vi "CAN_OBD仿真器.vi"() -> ()   [LabVIEW 2018]
doc: "This example demonstrates frame streaming input using an NI-XNET Frame Input session. \n\nThis example can run against any output example, assuming you have a properly terminated CAN cable connected to two CAN ports.\n\nIf you have no database aliases on your system, the example automatically loads the nixnet_example database."
uses:
  <vilib>/xnet/xnet.llb/XNET Frame CAN.ctl
  <vilib>/xnet/xnet.llb/XNET Frame Type CAN.ctl
  <vilib>/xnet/xnet.llb/XNET Create Session (Frame Input Stream).vi
  <vilib>/xnet/xnet.llb/XNET Create Session (Frame Output Stream).vi
  <vilib>/xnet/xnet.llb/XNET Read (Frame CAN).vi
  <vilib>/xnet/xnet.llb/XNET Write (Frame CAN).vi
  <resource>/objmgr/xnet.rc
panel:
  in  "车速":u8(slide) scale=0.0..255.0
  in  "引擎转速":u16(slide) scale=0.0..20000.0
  out "data":T1[](array[typedef]) {"payload" format="%x"; "timestamp" format="%<%.7X\n%x>T"; "type" items=["CAN Data"=0, "CAN Remote"=1, "CAN Bus Error"=2, "CAN 2.0 Data"=8, "CAN FD Data"=16, "CAN FD+BRS Data"=24, "J1939 Data"=192, "Delay"=224, "Log Trigger"=225, "Start Trigger"=226]; "identifier" format="%x"}
  in  "Number of Frames to Display":i32=15
  in  "Hex Display":bool=TRUE
  in  "BaudRate":u32=500000
  out "Frames":string[][](table)
  in  "Select Interface":refnum<k21>="CAN2"
  in  "stop":bool
  # "Overview: Demonstrates the use of the CAN streaming frame input session.\nRequirements: LabVIEW, NI-XNET\nInstructions:\n1. Ensure that you are have connected the selected CAN port to another CAN interface outputting data. This example can be used with any CAN output example.\n2. Run the VI"
  # "If a cluster is selected, the cluster's baudrate will be used.  If the :memory: cluster is selected, a baudrate must be provided."
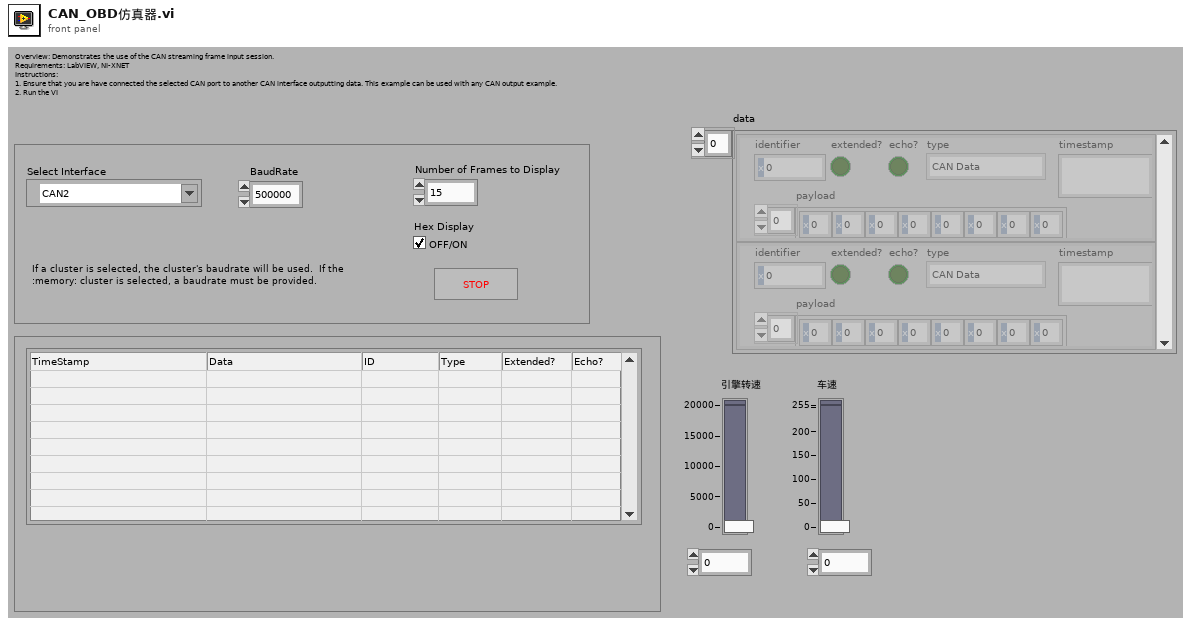
[diagram p1: front panel]
types:
  T1 = typedef "XNET Frame CAN.ctl" = cluster{"timestamp":timestamp, "payload":u8[], "identifier":u32, "type":T2, "extended?":bool, "echo?":bool}
  T2 = typedef "XNET Frame Type CAN.ctl" = u8
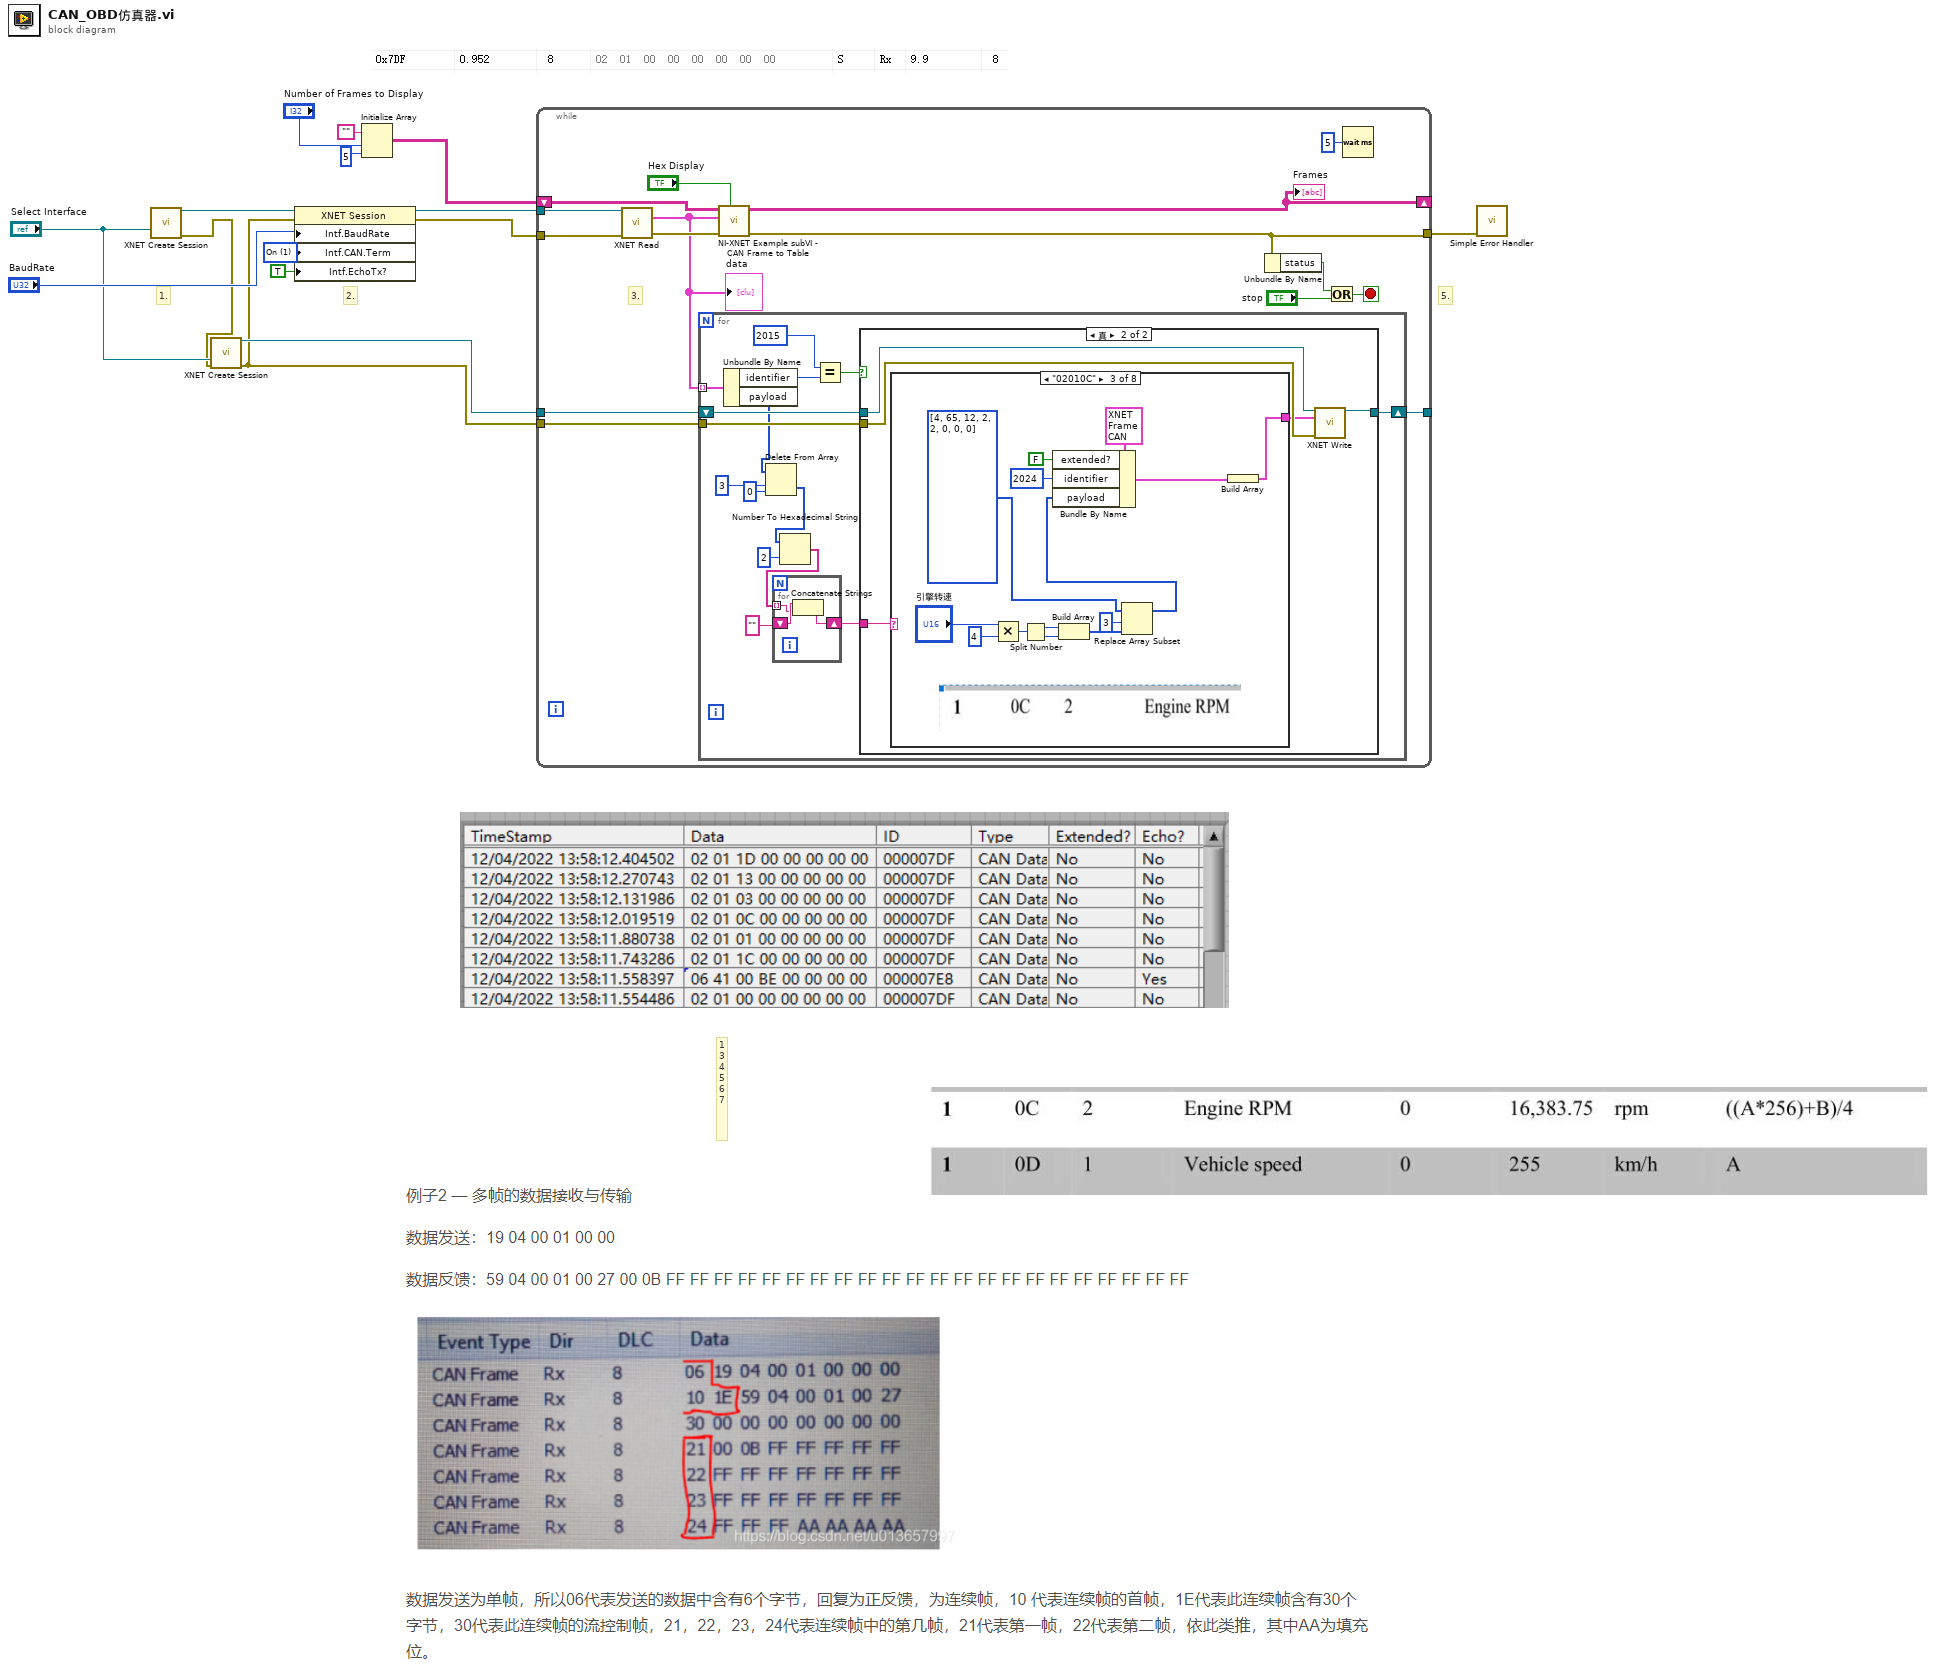
[diagram p0: block diagram]
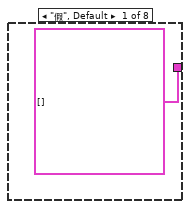
[diagram p3: hidden frame]
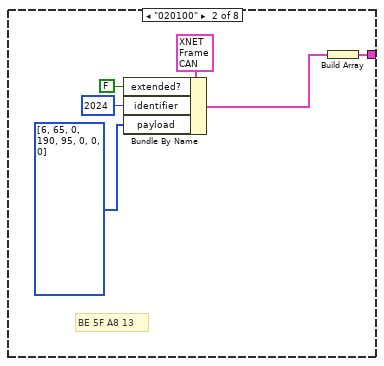
[diagram p4: hidden frame]
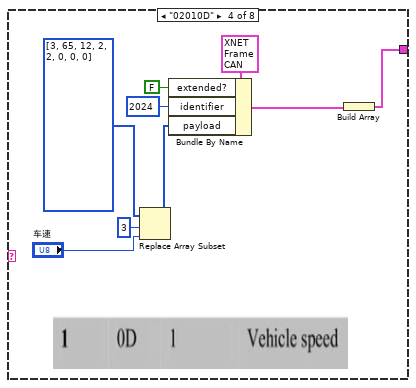
[diagram p5: hidden frame]
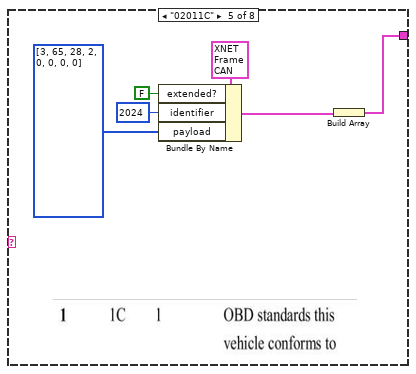
[diagram p6: hidden frame]
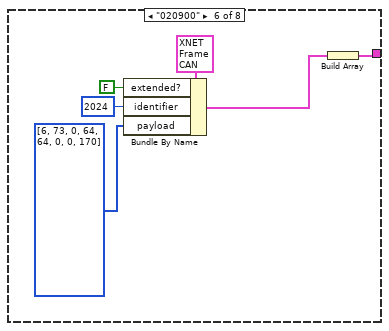
[diagram p7: hidden frame]
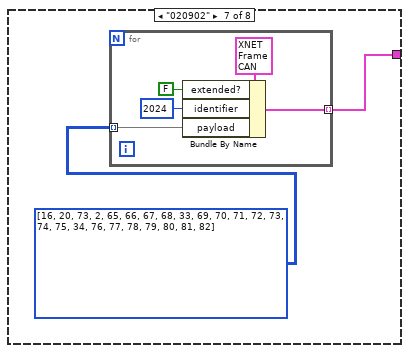
[diagram p8: hidden frame]
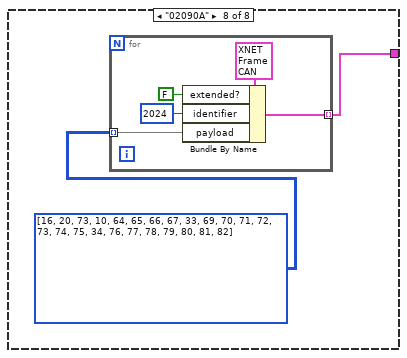
[diagram p9: hidden frame]
diagram:
  w6 = u32 1 items=["Off", "On"] ("Interface:CAN:Termination")
  # "1\n3\n4\n5\n6\n7"
  # "2."
  # "5."
  # "1."
  n1 = call-poly <vilib>:"XNET Create Session.vi"("interface"="Select Interface") -> ("session out"=w14:refnum<k21>, "error out"=w4:errorcluster)  [unwired: 2 in, 11 out]
  n2 = call-poly <vilib>:"XNET Create Session.vi"("interface"="Select Interface", "error in (no error)"=w4) -> ("session out"=w3:refnum<k21>, "error out"=w2:errorcluster)  [unwired: 1 in, 11 out]
  n3 = property class="XNET Session"(reference=w14, error in=w2, "Intf.BaudRate"="BaudRate", "Intf.CAN.Term"=w6, "Intf.EchoTx?"=TRUE ("Interface:Echo Transmit?")) -> (reference out=w13:refnum<k21>, error out=w11:errorcluster)
  n4 = Initialize Array("", "Number of Frames to Display", 5 ("Dimension Size")) -> (w7:string[][])
  n5 = while {
    tunnel: w13 -> [w30]
    tunnel: w11 -> [w29]
    tunnel: [w22] -> w15
    shift-right: [w24] -> _
    shift-left: w7 -> [w25]
    tunnel: w3 -> [w18]
    tunnel: w2 -> [w17]
    tunnel: [w16] -> _
    stop <- w26 stop-if-true
    # "3."
    n6 = call-poly <vilib>:"XNET Read.vi"("session in"=w30, "error in (no error)"=w29) -> ("data"=w19:T1[], "error out"=w23:errorcluster)  [unwired: 12 out]
    "data" <- w19
    n7 = for {
      tunnel: w19 -> [w45] mode=indexing
      tunnel: w17 -> [w43]
      shift-right: [w42] -> w16
      shift-left: w18 -> [w44]
      n8 = Unbundle By Name(w45) -> ("identifier"=w40:u32, "payload"=w34:u8[])
      n9 = Delete From Array(array=w34, length=3 ("长度"), index=0 ("索引")) -> (deleted portion=w33:u8[])  [unwired: 1 out]
      n10 = Number To Hexadecimal String(1:i16 2 ("宽度(-)"), 2:w33) -> (0:w38:string[])
      n11 = for {
        shift-right: [w48] -> w35
        shift-left: "" -> [w47]
        tunnel: w38 -> [w46] mode=indexing
        n12 = Concatenate Strings(w47, w46) -> (w48:string)
      }
      n13 = Equal?(x=u32 2015 ("y"), y=w40) -> (x = y?=w41:bool)
      n14 = case shown="真" w41 {
        tunnel: w44 -> [w49 w50]
        tunnel: w43 -> [_ w54]
        tunnel: [w49 w51] -> w42
        tunnel: w35 -> [_ w53]
        frame False {
        }
        frame True {
          n15 = case shown="\"02010C\"" w53 {
            tunnel: [T1[] [] w56 w71 w80 w86 w91 w98 w104] -> w52
            frame "假", Default {
            }
            frame "020100" {
              # "BE 5F A8 13"
              n16 = Bundle By Name(cluster=T1 {"timestamp"=timestamp(0 s since 1904-01-01), "payload"=[], "identifier"=0, "type"=0, "extended?"=FALSE, "echo?"=FALSE} ("CAN frame"), "extended?"=FALSE, "identifier"=u32 2024, "payload"=u8[] [6, 65, 0, 190, 95, 0, 0, 0]) -> (w60:T1)
              n17 = Build Array(w60) -> (w56:T1[])
            }
            frame "02010C" {
              n18 = Multiply(x="引擎转速", y=u16 4) -> (x*y=w69:u16)
              n19 = Split Number(x=w69) -> (hi(x)=w68:u8, lo(x)=w67:u8)
              n20 = Build Array(w68, w67) -> (w66:u8[])
              n21 = Replace Array Subset(array=u8[] [4, 65, 12, 2, 2, 0, 0, 0] ("payload"), new element=w66, index=3 ("索引")) -> (w62:u8[])
              n22 = Bundle By Name(cluster=T1 {"timestamp"=timestamp(0 s since 1904-01-01), "payload"=[], "identifier"=0, "type"=0, "extended?"=FALSE, "echo?"=FALSE} ("CAN frame"), "extended?"=FALSE, "identifier"=u32 2024, "payload"=w62) -> (w72:T1)
              n23 = Build Array(w72) -> (w71:T1[])
            }
            frame "02010D" {
              n24 = Replace Array Subset(array=u8[] [3, 65, 12, 2, 2, 0, 0, 0] ("payload"), new element="车速", index=3 ("索引")) -> (w76:u8[])
              n25 = Bundle By Name(cluster=T1 {"timestamp"=timestamp(0 s since 1904-01-01), "payload"=[], "identifier"=0, "type"=0, "extended?"=FALSE, "echo?"=FALSE} ("CAN frame"), "extended?"=FALSE, "identifier"=u32 2024, "payload"=w76) -> (w81:T1)
              n26 = Build Array(w81) -> (w80:T1[])
            }
            frame "02011C" {
              n27 = Bundle By Name(cluster=T1 {"timestamp"=timestamp(0 s since 1904-01-01), "payload"=[], "identifier"=0, "type"=0, "extended?"=FALSE, "echo?"=FALSE} ("CAN frame"), "extended?"=FALSE, "identifier"=u32 2024, "payload"=u8[] [3, 65, 28, 2, 0, 0, 0, 0]) -> (w87:T1)
              n28 = Build Array(w87) -> (w86:T1[])
            }
            frame "020900" {
              n29 = Bundle By Name(cluster=T1 {"timestamp"=timestamp(0 s since 1904-01-01), "payload"=[], "identifier"=0, "type"=0, "extended?"=FALSE, "echo?"=FALSE} ("CAN frame"), "extended?"=FALSE, "identifier"=u32 2024, "payload"=u8[] [6, 73, 0, 64, 64, 0, 0, 170]) -> (w95:T1)
              n30 = Build Array(w95) -> (w91:T1[])
            }
            frame "020902" {
              n31 = for {
                tunnel: [w100] -> w98 mode=indexing
                tunnel: u8[][] [[16, 20, 73, 2, 65, 66, 67, 68], [33, 69, 70, 71, 72, 73, 74, 75], [34, 76, 77, 78, 79, 80, 81, 82]] ("payload") -> [w99] mode=indexing
                n32 = Bundle By Name(cluster=T1 {"timestamp"=timestamp(0 s since 1904-01-01), "payload"=[], "identifier"=0, "type"=0, "extended?"=FALSE, "echo?"=FALSE} ("CAN frame"), "extended?"=FALSE, "identifier"=u32 2024, "payload"=w99) -> (w100:T1)
              }
            }
            frame "02090A" {
              n33 = for {
                tunnel: [w107] -> w104 mode=indexing
                tunnel: u8[][] [[16, 20, 73, 10, 64, 65, 66, 67], [33, 69, 70, 71, 72, 73, 74, 75], [34, 76, 77, 78, 79, 80, 81, 82]] ("payload") -> [w106] mode=indexing
                n34 = Bundle By Name(cluster=T1 {"timestamp"=timestamp(0 s since 1904-01-01), "payload"=[], "identifier"=0, "type"=0, "extended?"=FALSE, "echo?"=FALSE} ("CAN frame"), "extended?"=FALSE, "identifier"=u32 2024, "payload"=w106) -> (w107:T1)
              }
            }
          }
          n35 = call-poly <vilib>:"XNET Write.vi"("session in"=w50, "data"=w52, "error in (no error)"=w54) -> ("session out"=w51:refnum<k21>)  [unwired: 12 out]
        }
      }
    }
    n36 = call "NI-XNET Example subVI - CAN Frame to Table.vi"("Hexadecimal?"="Hex Display", "error in (no error)"=w23, "CAN Frames (from XNET Read)"=w19, "Input Array"=w25) -> ("error out"=w22:errorcluster, "Output Array"=w24:string[][])  [unwired: 1 in, 5 out]
    "Frames" <- w24
    n37 = Unbundle By Name(w22) -> ("status"=w28:bool)
    n38 = Or(x=w28, y="stop") -> (x .or. y?=w26:bool)
    n39 = Wait (ms)(milliseconds to wait=u32 5) -> ()  [unwired: 1 out]
  }
  n40 = call <vilib>:"Simple Error Handler.vi"("error in (no error)"=w15) -> ()  [unwired: 1 in, 8 out]
